vi "ICM Create String.vi"(0 "Data":T1(array[cluster]), 3 "Current Position":i32) -> (7 "String Out":string)   [LabVIEW 2024]
doc: "OSDS Create String.vi\n\n This VI is used by the OSDS Simulator to create a frame string, either from recorded data or by creating simulated data.\n\nOCC Streaming Data System Version 1.0\nJune, 2007 Original Code Consulting David Thomson\n www.originalcode.com"
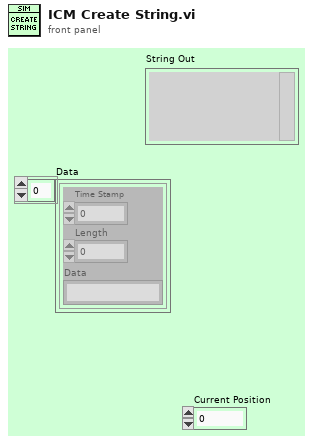
[diagram p1: front panel]
types:
  T1 = cluster{"Time Stamp":dbl, "Length":i32, "Data":string}[]
  T2 = cluster{"Time Stamp":dbl, "Length":i32, "Data":string}
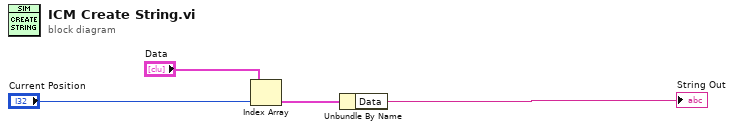
[diagram p0: block diagram]
diagram:
  n1 = Index Array(array="Data", index="Current Position") -> (element=w1:T2)
  n2 = Unbundle By Name(w1) -> ("Data"=→"String Out":string)
